vi "Process File.vi"(8 "error in (no error)":errorcluster, 10 "File":path, 11 "Lockin Processor in":refnum<class "Lockin Processor.lvclass">) -> (0 "error out":errorcluster, 2 "File out":path, 3 "Lockin Processor out":refnum<class "Lockin Processor.lvclass">)   [LabVIEW 2016, in "Lockin Processor.lvclass"]
uses:
  Lockin Processor.lvclass
  Lockin Processor.lvclass/Lockin Processor.ctl
  Read Lockin Processor Configuration.vi
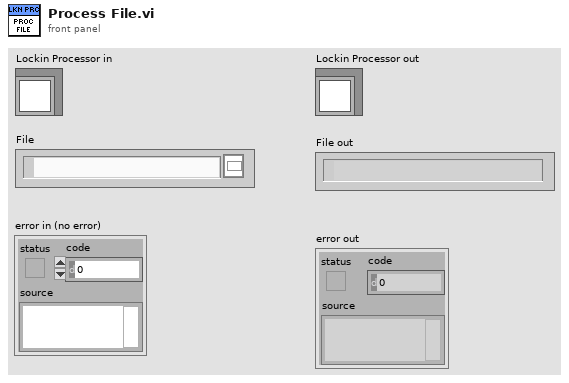
[diagram p1: front panel]
types:
  T1 = typedef "Lockin Processor Configuration.ctl" = cluster{"Time constant":dbl, "Phase":dbl, "Signal channels":string[], "Group":string, "X channel":string, "Live update":bool}
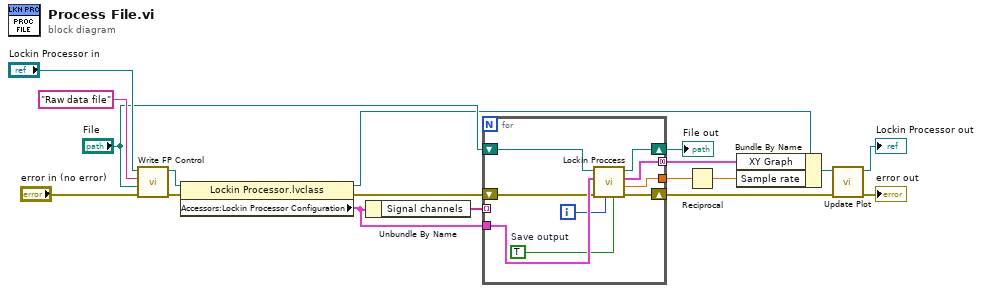
[diagram p0: block diagram]
diagram:
  n1 = call-dynamic "Write FP Control.vi"("error in (no error)"="error in (no error)", "Control Value"="File", "Control Name"="Raw data file", "Measure Object in"="Lockin Processor in") -> ("error out"=w13:errorcluster, "Measure Object out"=w15:refnum<class "Lockin Processor.lvclass">)  [unwired: 6 in]
  n2 = property class="Lockin Processor.lvclass"(reference=w15, error in=w13) -> (reference out=w8:refnum<class "Lockin Processor.lvclass">, error out=w17:errorcluster, "Accessors:Lockin Processor Configuration"=w12:T1)
  n3 = Unbundle By Name(w12) -> ("Signal channels"=w11:string[])
  n4 = for {
    shift-right: [w21] -> w9
    shift-left: "File" -> [w22]
    shift-right: [w23] -> w4
    shift-left: w17 -> [w24]
    tunnel: w12 -> [w27]
    tunnel: w11 -> [_] mode=indexing
    tunnel: [w20] -> w7 mode=concatenating
    tunnel: [w19] -> w2
    i -> [w25]
    w26 = TRUE  # Save output
    n5 = call "Lockin Proccess.vi"("Save output"=w26, "CH index"=w25, "Error In"=w24, "User configuration"=w27, "Signal file"=w22) -> ("Error Out"=w23:errorcluster, "dt"=w19:dbl, "XY Graph"=w20:cluster{dbl[], "Y":dbl[]}[], "Signal file out"=w21:path)  [unwired: 3 in]
  }
  "File out" <- w9
  n6 = Reciprocal(x=w2) -> (1/x=w1:dbl)
  n7 = Bundle By Name(cluster=w8, "XY Graph"=w7, "Sample rate"=w1) -> (w6:refnum<class "Lockin Processor.lvclass">)
  n8 = call-dynamic "Update Plot.vi"("error in (no error)"=w4, "Lockin Processor in"=w6) -> ("error out"=→"error out":errorcluster, "Lockin Processor out"=→"Lockin Processor out":refnum<class "Lockin Processor.lvclass">)  [unwired: 8 in]
